vi "Get centroid.vi"(1 "V2":sgl[](array[numeric]), 2 "V1":sgl[](array[numeric]), 3 "V0":sgl[](array[numeric]), 4 "Centroid type":u8(ring) items=["Centroid", "Barycenter", "Random"]) -> (0 "Pc":sgl[](array[numeric]))   [LabVIEW 2017]
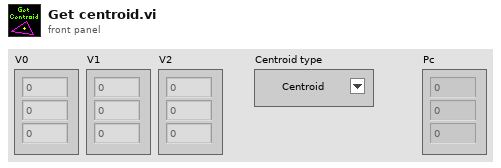
[diagram p1: front panel]
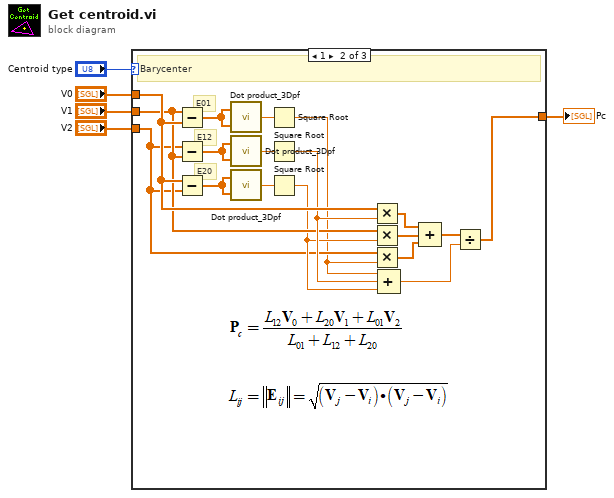
[diagram p0: block diagram]
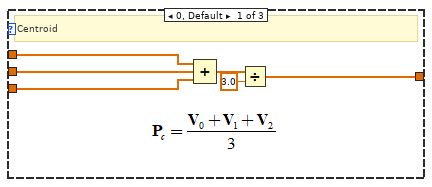
[diagram p2: hidden frame]
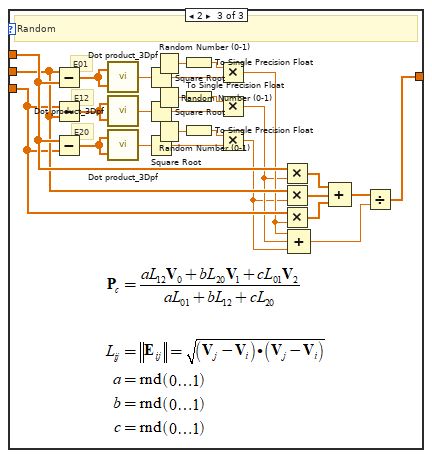
[diagram p3: hidden frame]
diagram:
  n1 = case shown="1" "Centroid type" {
    tunnel: "V0" -> [w9 w23 w50]
    tunnel: "V1" -> [w8 w21 w49]
    tunnel: "V2" -> [w7 w19 w48]
    tunnel: [w6 w12 w42] -> w1
    frame 0, Default {
      # "Centroid"
      n2 = Compound Arithmetic op=ADD(w9, w8, w7) -> (w11:sgl[])
      n3 = Divide(x=w11, y=sgl 3.0 ("Numeric")) -> (x/y=w6:sgl[])
    }
    frame 1 {
      # "E20"
      # "E12"
      # "E01"
      # "Barycenter"
      n4 = Subtract(x=w21, y=w23) -> (x-y=w29:sgl[])
      n5 = Subtract(x=w19, y=w21) -> (x-y=w28:sgl[])
      n6 = Subtract(x=w23, y=w19) -> (x-y=w27:sgl[])
      n7 = call "Dot product_3Dpf.vi"("B"=w29, "A"=w29) -> ("A . B"=w26:sgl)
      n8 = call "Dot product_3Dpf.vi"("B"=w28, "A"=w28) -> ("A . B"=w25:sgl)
      n9 = call "Dot product_3Dpf.vi"("B"=w27, "A"=w27) -> ("A . B"=w24:sgl)
      n10 = Square Root(x=w26) -> (sqrt(x)=w18:sgl)
      n11 = Square Root(x=w25) -> (sqrt(x)=w22:sgl)
      n12 = Square Root(x=w24) -> (sqrt(x)=w20:sgl)
      n13 = Multiply(x=w23, y=w22) -> (x*y=w17:sgl[])
      n14 = Multiply(x=w21, y=w20) -> (x*y=w16:sgl[])
      n15 = Multiply(x=w19, y=w18) -> (x*y=w15:sgl[])
      n16 = Compound Arithmetic op=ADD(w18, w22, w20) -> (w13:sgl)
      n17 = Compound Arithmetic op=ADD(w17, w16, w15) -> (w14:sgl[])
      n18 = Divide(x=w14, y=w13) -> (x/y=w12:sgl[])
    }
    frame 2 {
      # "E20"
      # "E12"
      # "E01"
      # "Random"
      n19 = Subtract(x=w49, y=w50) -> (x-y=w56:sgl[])
      n20 = Subtract(x=w48, y=w49) -> (x-y=w55:sgl[])
      n21 = Subtract(x=w50, y=w48) -> (x-y=w54:sgl[])
      n22 = call "Dot product_3Dpf.vi"("B"=w56, "A"=w56) -> ("A . B"=w53:sgl)
      n23 = call "Dot product_3Dpf.vi"("B"=w55, "A"=w55) -> ("A . B"=w52:sgl)
      n24 = call "Dot product_3Dpf.vi"("B"=w54, "A"=w54) -> ("A . B"=w51:sgl)
      n25 = Square Root(x=w53) -> (sqrt(x)=w40:sgl)
      n26 = Square Root(x=w52) -> (sqrt(x)=w37:sgl)
      n27 = Square Root(x=w51) -> (sqrt(x)=w34:sgl)
      n28 = Random Number (0-1)() -> (number: 0 to 1=w41:dbl)
      n29 = Random Number (0-1)() -> (number: 0 to 1=w38:dbl)
      n30 = Random Number (0-1)() -> (number: 0 to 1=w35:dbl)
      n31 = To Single Precision Float(number=w41) -> (single precision float=w32:sgl)
      n32 = To Single Precision Float(number=w38) -> (single precision float=w31:sgl)
      n33 = To Single Precision Float(number=w35) -> (single precision float=w30:sgl)
      n34 = Multiply(x=w32, y=w40) -> (x*y=w39:sgl)
      n35 = Multiply(x=w31, y=w37) -> (x*y=w36:sgl)
      n36 = Multiply(x=w30, y=w34) -> (x*y=w33:sgl)
      n37 = Multiply(x=w50, y=w36) -> (x*y=w47:sgl[])
      n38 = Multiply(x=w49, y=w33) -> (x*y=w46:sgl[])
      n39 = Multiply(x=w48, y=w39) -> (x*y=w45:sgl[])
      n40 = Compound Arithmetic op=ADD(w39, w36, w33) -> (w43:sgl)
      n41 = Compound Arithmetic op=ADD(w47, w46, w45) -> (w44:sgl[])
      n42 = Divide(x=w44, y=w43) -> (x/y=w42:sgl[])
    }
  }
  "Pc" <- w1
